vi "3D Graph (SubVI).vi"(1 "Interpolate":i32, 3 "error in (no error)":errorcluster, 4 "Z":dbl, 5 "Y":dbl, 6 "X":dbl) -> (0 "error out":errorcluster, 2 "3D Plot lvclass Array out":refnum<class "3D Plot Datatype.lvclass">[](array[class]))   [LabVIEW 2012]
uses:
  <vilib>/Math Plots/3D Math Plots/3D Plot/3D Plot Datatype/3D Plot Datatype.lvclass
  <vilib>/Math Plots/3D Math Plots/3D Scatter/3D Scatter Datatype/Public/Plot Helper (Vector).vi
  <vilib>/Math Plots/3D Math Plots/3D Scatter/3D Scatter Datatype/3D Scatter Datatype.lvclass
panel:
  out "Interpolated Array":dbl[](array[numeric])
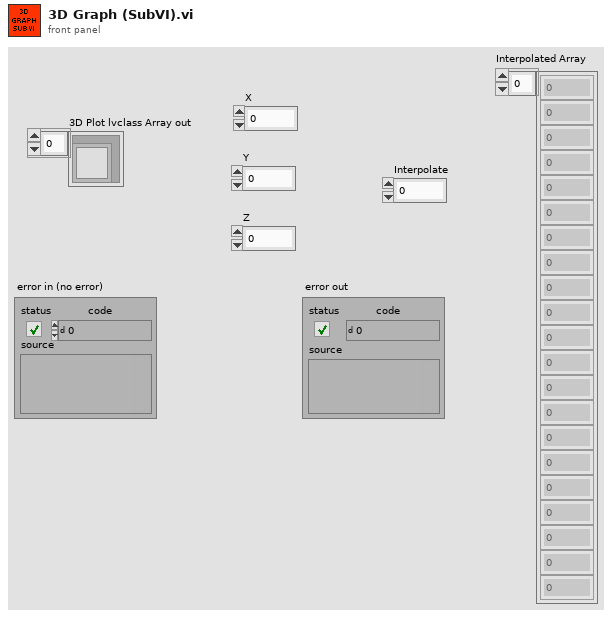
[diagram p1: front panel]
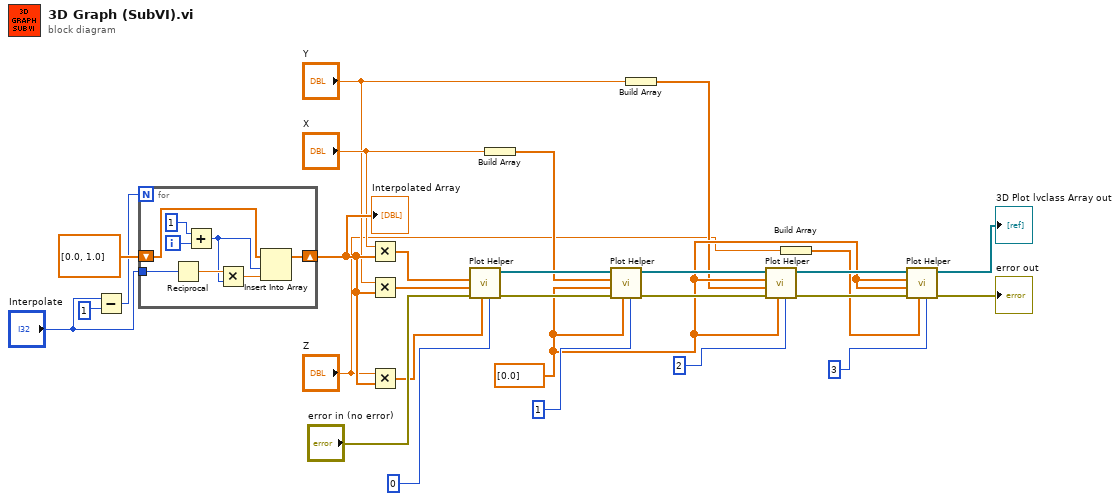
[diagram p0: block diagram]
diagram:
  w7 = sgl[] [0.0] ("y vector")
  n1 = Subtract(x="Interpolate", y=1) -> (x-y=w11:i32)
  n2 = for {
    N: w11 -> [_]
    shift-right: [w33] -> w9
    shift-left: dbl[] [0.0, 1.0] ("array of numbers or points") -> [w36]
    tunnel: "Interpolate" -> [w32]
    i -> [w31]
    n3 = Reciprocal(x=w32) -> (1/x=w35:dbl)
    n4 = Add(x=1, y=w31) -> (x+y=w29:i32)
    n5 = Multiply(x=w35, y=w29) -> (x*y=w34:dbl)
    n6 = Insert Into Array(array=w36, index=w29, new element=w34) -> (w33:dbl[])
  }
  "Interpolated Array" <- w9
  n7 = Multiply(x="X", y=w9) -> (x*y=w20:dbl[])
  n8 = Multiply(x="Y", y=w9) -> (x*y=w19:dbl[])
  n9 = Multiply(x="Z", y=w9) -> (x*y=w18:dbl[])
  n10 = call-poly <vilib>:"Plot Helper.vi"("Plot ID"=0, "z vector"=w18, "error in (no error)"="error in (no error)", "y vector"=w19, "x vector"=w20) -> ("error out"=w26:errorcluster, "3D Plot lvclass Array out"=w27:refnum<class "3D Plot Datatype.lvclass">[])  [unwired: 1 in, 4 out]
  n11 = Build Array("X") -> (w5:dbl[])
  n12 = call-poly <vilib>:"Plot Helper.vi"("Plot ID"=1, "z vector"=w7, "error in (no error)"=w26, "y vector"=w7, "x vector"=w5, "3D Plot lvclass Array in"=w27) -> ("error out"=w25:errorcluster, "3D Plot lvclass Array out"=w24:refnum<class "3D Plot Datatype.lvclass">[])  [unwired: 4 out]
  n13 = Build Array("Y") -> (w3:dbl[])
  n14 = call-poly <vilib>:"Plot Helper.vi"("Plot ID"=2, "z vector"=w7, "error in (no error)"=w25, "y vector"=w3, "x vector"=w7, "3D Plot lvclass Array in"=w24) -> ("error out"=w21:errorcluster, "3D Plot lvclass Array out"=w22:refnum<class "3D Plot Datatype.lvclass">[])  [unwired: 4 out]
  n15 = Build Array("Z") -> (w2:dbl[])
  n16 = call-poly <vilib>:"Plot Helper.vi"("Plot ID"=3, "z vector"=w2, "error in (no error)"=w21, "y vector"=w7, "x vector"=w7, "3D Plot lvclass Array in"=w22) -> ("error out"=→"error out":errorcluster, "3D Plot lvclass Array out"=→"3D Plot lvclass Array out":refnum<class "3D Plot Datatype.lvclass">[])  [unwired: 4 out]
